vi "speedcontrol1old.vi"(11 "queue in":refnum<queue>) -> ()   [LabVIEW 2014]
uses:
  controls/UI Data.ctl
  controls/EncoderController.ctl
  <vilib>/Platform/TimedLoop/XDataNode/timing_clust.ctl
  <vilib>/Platform/TimedLoop/XDataNode/nitl_modes.ctl
  <vilib>/Platform/TimedLoop/XDataNode/wakeup.ctl
  controls/Control StateSam.ctl
  controls/Control ConfigurationSam.ctl
  <vilib>/Platform/TimedLoop/XDataNode/loadnilvce.vi
  <vilib>/addons/control/pid/pid.llb/PID (DBL Array).vi
  <vilib>/addons/control/pid/pid.llb/PID Percentage to EGU (DBL Array).vi
  <vilib>/platform/TimedLoop/XDataNode/XDataNode.xnode
  <vilib>/addons/control/pid/NI_PID_pid.lvlib
  <vilib>/Platform/TimedLoop/XDataNode/XDNodeRunTimeDep.lvlib
panel:
  out "Motor3Output":dbl
  out "Motor2Output":dbl
  out "Velocity3 RPM":dbl
  out "Velocity2 RPM":dbl
  out "Motor4Output":dbl
  out "Velocity4 RPM":dbl
  out "Motor1Output":dbl
  out "Velocity1 RPM":dbl
  # "0.8, 0. 0 is stable but theres a large offset\nsystem is slow to settle, increase Ti"
  # "Kp=2.04, Ti=0.15, Td=0.0375"
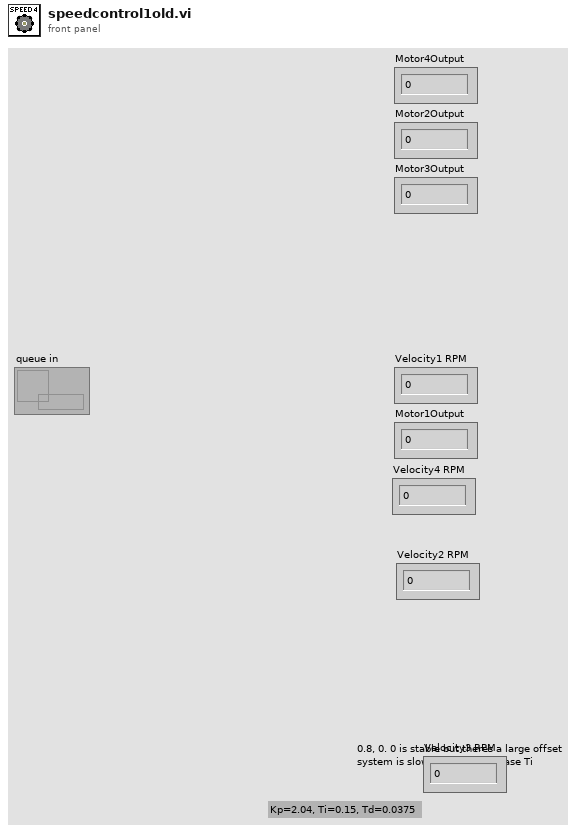
[diagram p1: front panel]
types:
  T1 = cluster{bool, "Tick Count(uSec)":u32, "Counter Value":i32, "x-y":i32}
  T2 = typedef "XDNodeRunTimeDep.lvlib/timing_clust.ctl" = cluster{"Expected End [f-1]":u64, "Actual End [f-1]":u64, "Finished Late? [f-1]":bool, "Expected End [i-1]":u64, "Actual End [i-1]":u64, "Finished Late? [i-1]":bool, "Expected Start [i]":u64, "Actual Start [i]":u64, "Expected Start [f]":u64, "Actual Start [f]":u64, "Source Name":string, "Structure Name":string, "Period":i64, "Deadline":i64, "Offset":i64, "Start":i64, "Priority":i32, "Timeout":i32, "Mode":T3, "Wakeup Reason":T4, "Error":errorcluster, "Source Type":string, "Secondary Source Type":string, "Global End Time":u64, "Global Start Time":u64, "Frame Duration":u64, "Iteration Duration":u64, "Assigned CPU":i32, "I/O Scan Engine Mode":u32}
  T3 = typedef "XDNodeRunTimeDep.lvlib/nitl_modes.ctl" = enum32{"No Change", "Process missed periods, maintain original phase", "Discard missed periods, maintain original phase", "Process missed periods, ignore original phase", "Discard missed periods, ignore original phase"}
  T4 = typedef "XDNodeRunTimeDep.lvlib/wakeup.ctl" = enum32{"Normal", "Aborted", "Asynchronous wakeup", "Timing source error", "Timed loop error", "Timeout"}
  T5 = typedef "EncoderController.ctl" = cluster{"Sample time (uS)":u32, "Reset":bool}
  T6 = typedef "EncoderIndicator.ctl" = cluster{"Position":dbl, "Velocity RPM":dbl, "Velocity RPS":dbl}
  T7 = typedef "Control StateSam.ctl" = enum16{"", "Control State (PID)", "Safe State"}
  T8 = typedef "Control ConfigurationSam.ctl" = cluster{"PID Gains":cluster{"proportional gain (Kc)":dbl, "integral gain (Kc*Ts/Ti)":dbl, "derivative gain (Kc*Td/Ts)":dbl}, "Output Range":cluster{"output high":dbl, "output low":dbl}}
  T9 = cluster{"proportional gain (Kc)":dbl, "integral gain (Kc*Ts/Ti)":dbl, "derivative gain (Kc*Td/Ts)":dbl}[]
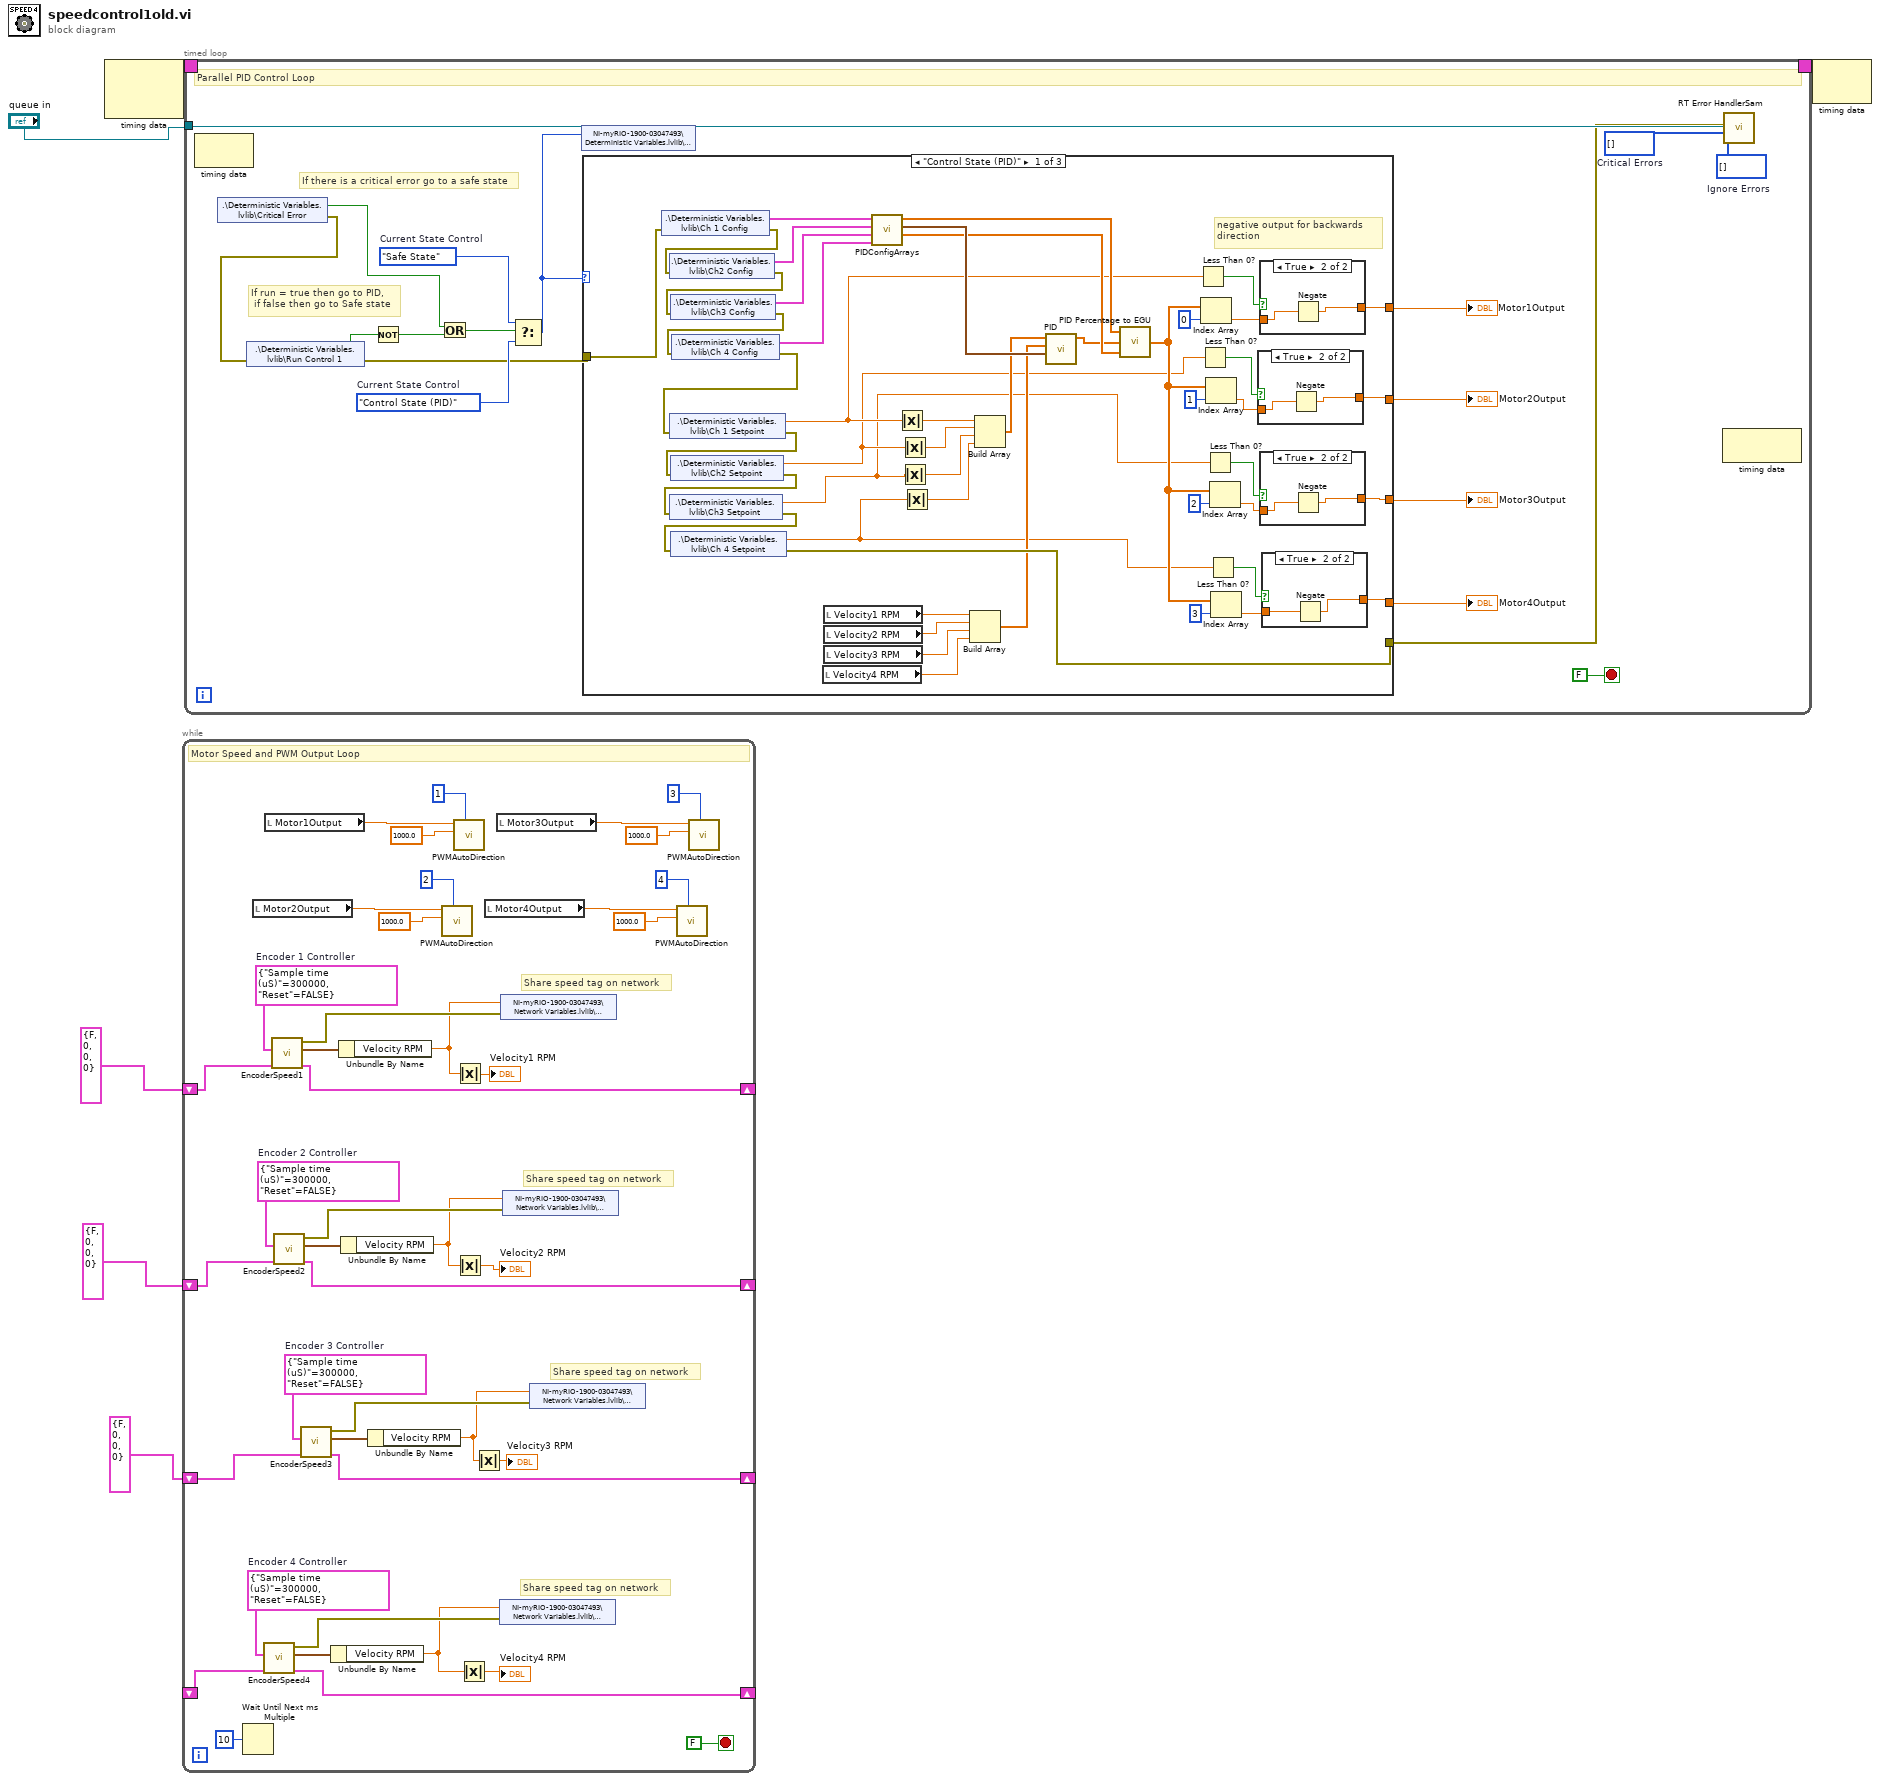
[diagram p0: block diagram]
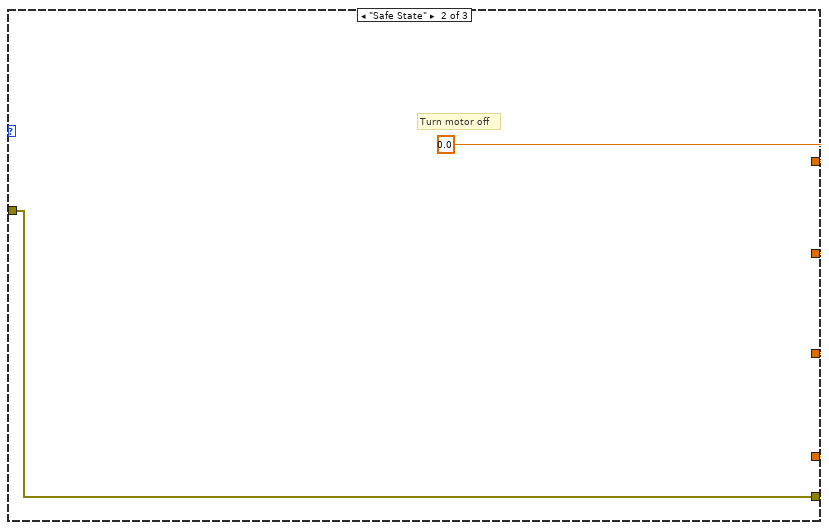
[diagram p6: hidden frame]
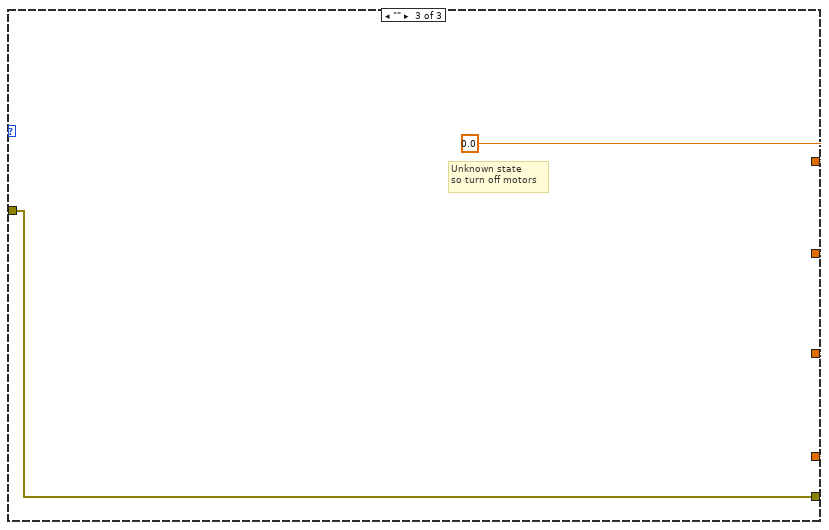
[diagram p7: hidden frame]
diagram:
  n1 = node-c288() -> (w6:T2)  [unwired: 2 in]
  n2 = while {
    shift-right: [w44] -> _
    shift-left: T1 {FALSE, "Tick Count(uSec)"=0, "Counter Value"=0, "x-y"=0} ("Cluster out") -> [w45]
    shift-right: [w34] -> _
    shift-left: _ -> [w35]
    shift-right: [w30] -> _
    shift-left: T1 {FALSE, "Tick Count(uSec)"=0, "Counter Value"=0, "x-y"=0} ("Cluster out") -> [w29]
    shift-right: [w21] -> _
    shift-left: T1 {FALSE, "Tick Count(uSec)"=0, "Counter Value"=0, "x-y"=0} ("Cluster out") -> [w22]
    stop <- FALSE stop-if-true
    w25 = T5 {"Sample time (uS)"=300000, "Reset"=FALSE}  # Encoder 3 Controller
    w26 = T5 {"Sample time (uS)"=300000, "Reset"=FALSE}  # Encoder 2 Controller
    w36 = T5 {"Sample time (uS)"=300000, "Reset"=FALSE}  # Encoder 4 Controller
    w48 = T5 {"Sample time (uS)"=300000, "Reset"=FALSE}  # Encoder 1 Controller
    # "Share speed tag on network"
    # "Share speed tag on network"
    # "Share speed tag on network"
    # "Share speed tag on network"
    # "Motor Speed and PWM Output Loop"
    n3 = Wait Until Next ms Multiple(millisecond multiple=u32 10) -> ()  [unwired: 1 out]
    n4 = local read "Motor2Output"() -> (w15:dbl)
    n5 = call "EncoderSpeed4.vi"("Cluster in"=w35, "Encoder 4 Controller"=w36) -> ("Cluster out"=w34:T1, "Encoder 4 Indicator"=w37:T6, "error out"=w38:errorcluster)  [unwired: 7 in]
    n6 = local read "Motor1Output"() -> (w41:dbl)
    n7 = call "EncoderSpeed1.vi"("Cluster in"=w45, "Encoder 1 Controller"=w48) -> ("Cluster out"=w44:T1, "Encoder 1 Indicator"=w47:T6, "error out"=w46:errorcluster)  [unwired: 7 in]
    n8 = call "EncoderSpeed2.vi"("Cluster in"=w29, "Encoder 2 Controller"=w26) -> ("Cluster out"=w30:T1, "Encoder 2 Indicator"=w27:T6, "error out"=w28:errorcluster)  [unwired: 7 in]
    n9 = call "EncoderSpeed3.vi"("Cluster in"=w22, "Encoder 3 Controller"=w25) -> ("Cluster out"=w21:T1, "Encoder 3 Indicator"=w24:T6, "error out"=w23:errorcluster)  [unwired: 7 in]
    n10 = Unbundle By Name(w37) -> ("Velocity RPM"=w7:dbl)
    n11 = Unbundle By Name(w47) -> ("Velocity RPM"=w13:dbl)
    n12 = Unbundle By Name(w27) -> ("Velocity RPM"=w12:dbl)
    n13 = Unbundle By Name(w24) -> ("Velocity RPM"=w10:dbl)
    n14 = call "PWMAutoDirection.vi"("Motor Select"=i8 2, "PWM Frequency"=1000.0, "DutyCycle"=w15) -> ()  [unwired: 8 in, 1 out]
    n15 = call "PWMAutoDirection.vi"("Motor Select"=i8 1, "PWM Frequency"=1000.0, "DutyCycle"=w41) -> ()  [unwired: 8 in, 1 out]
    n16 = Absolute Value(x=w13) -> (abs(x)=→"Velocity1 RPM":dbl)
    n17 = Absolute Value(x=w12) -> (abs(x)=→"Velocity2 RPM":dbl)
    n18 = Absolute Value(x=w7) -> (abs(x)=→"Velocity4 RPM":dbl)
    n19 = Absolute Value(x=w10) -> (abs(x)=→"Velocity3 RPM":dbl)
    n20 = local read "Motor4Output"() -> (w20:dbl)
    n21 = local read "Motor3Output"() -> (w31:dbl)
    n22 = shared-variable "NI-myRIO-1900-03047493\\Network Variables.lvlib\\SpeedMotor4"(w7, error in=w38) -> ()  [unwired: 1 out]
    n23 = shared-variable "NI-myRIO-1900-03047493\\Network Variables.lvlib\\SpeedMotor1"(w13, error in=w46) -> ()  [unwired: 1 out]
    n24 = shared-variable "NI-myRIO-1900-03047493\\Network Variables.lvlib\\SpeedMotor2"(w12, error in=w28) -> ()  [unwired: 1 out]
    n25 = shared-variable "NI-myRIO-1900-03047493\\Network Variables.lvlib\\SpeedMotor3"(w10, error in=w23) -> ()  [unwired: 1 out]
    n26 = call "PWMAutoDirection.vi"("Motor Select"=i8 4, "PWM Frequency"=1000.0, "DutyCycle"=w20) -> ()  [unwired: 8 in, 1 out]
    n27 = call "PWMAutoDirection.vi"("Motor Select"=i8 3, "PWM Frequency"=1000.0, "DutyCycle"=w31) -> ()  [unwired: 8 in, 1 out]
  }
  n28 = timed-loop {
    timing: w6 -> [_]
    timing-out: [_] -> w5
    tunnel: "queue in" -> [w54]
    stop <- FALSE stop-if-true
    w55 = i32[] []  # Critical Errors
    w56 = i32[] []  # Ignore Errors
    w63 = Control_StateSam."Control State (PID)"  # Current State Control
    w64 = Control_StateSam."Safe State"  # Current State Control
    # "If there is a critical error go to a safe state"
    # "If run = true then go to PID,\n if false then go to Safe state"
    # "Parallel PID Control Loop"
    n29 = node-c288() -> ()  [unwired: 1 in, 1 out]
    n30 = shared-variable ".\\Deterministic Variables.lvlib\\Critical Error"() -> (w60:bool, error out=w58:errorcluster)  [unwired: 1 in]
    n31 = shared-variable ".\\Deterministic Variables.lvlib\\Run Control 1"(error in=w58) -> (w65:bool, error out=w57:errorcluster)
    n32 = Not(x=w65) -> (.not. x?=w61:bool)
    n33 = Or(x=w60, y=w61) -> (x .or. y?=w59:bool)
    n34 = Select(t=w64, s=w59, f=w63) -> (s? t:f=w62:T7)
    n35 = shared-variable "NI-myRIO-1900-03047493\\Deterministic Variables.lvlib\\Control State"(w62) -> ()  [unwired: 1 in, 1 out]
    n36 = case shown="\"Control State (PID)\"" w62 {
      tunnel: [w86 w127 w129] -> w53
      tunnel: w57 -> [w97 w128 w130]
      tunnel: [w114 w128 w130] -> w52
      tunnel: [w80 w127 w129] -> w51
      tunnel: [w81 w127 w129] -> w50
      tunnel: [w82 w127 w129] -> w49
      frame "Control State (PID)" {
        # "negative output for backwards \ndirection"
        n37 = shared-variable ".\\Deterministic Variables.lvlib\\Ch 1 Config"(error in=w97) -> (w113:T8, error out=w96:errorcluster)
        n38 = shared-variable ".\\Deterministic Variables.lvlib\\Ch2 Config"(error in=w96) -> (w112:T8, error out=w95:errorcluster)
        n39 = shared-variable ".\\Deterministic Variables.lvlib\\Ch3 Config"(error in=w95) -> (w93:T8, error out=w94:errorcluster)
        n40 = shared-variable ".\\Deterministic Variables.lvlib\\Ch 4 Config"(error in=w94) -> (w92:T8, error out=w89:errorcluster)
        n41 = shared-variable ".\\Deterministic Variables.lvlib\\Ch 1 Setpoint"(error in=w89) -> (w74:dbl, error out=w100:errorcluster)
        n42 = shared-variable ".\\Deterministic Variables.lvlib\\Ch2 Setpoint"(error in=w100) -> (w72:dbl, error out=w99:errorcluster)
        n43 = shared-variable ".\\Deterministic Variables.lvlib\\Ch3 Setpoint"(error in=w99) -> (w68:dbl, error out=w98:errorcluster)
        n44 = shared-variable ".\\Deterministic Variables.lvlib\\Ch 4 Setpoint"(error in=w98) -> (w71:dbl, error out=w114:errorcluster)
        n45 = local read "Velocity4 RPM"() -> (w101:dbl)
        n46 = local read "Velocity1 RPM"() -> (w105:dbl)
        n47 = local read "Velocity2 RPM"() -> (w104:dbl)
        n48 = local read "Velocity3 RPM"() -> (w102:dbl)
        n49 = call "PIDConfigArrays.vi"("CH4"=w92, "CH3"=w93, "CH2"=w112, "CH1"=w113) -> ("OR Low array"=w109:dbl[], "OR High array"=w110:dbl[], "PID Gains array"=w111:T9)  [unwired: 5 in]
        n50 = Absolute Value(x=w74) -> (abs(x)=w73:dbl)
        n51 = Absolute Value(x=w72) -> (abs(x)=w69:dbl)
        n52 = Absolute Value(x=w68) -> (abs(x)=w67:dbl)
        n53 = Absolute Value(x=w71) -> (abs(x)=w70:dbl)
        n54 = Build Array(w105, w104, w102, w101) -> (w103:dbl[])
        n55 = Build Array(w73, w69, w67, w70) -> (w106:dbl[])
        n56 = call-poly <vilib>:"PID.vi"("PID gains"=w111, "process variable"=w103, "setpoint"=w106) -> ("output"=w75:dbl[])  [unwired: 7 in, 1 out]
        n57 = call-poly <vilib>:"PID Percentage to EGU.vi"("minimum (EGU)"=w109, "% span"=w75, "maximum (EGU)"=w110) -> ("output (EGU)"=w90:dbl[])  [unwired: 1 in]
        n58 = Less Than 0?(x=w74) -> (x < 0?=w88:bool)
        n59 = Less Than 0?(x=w72) -> (x < 0?=w78:bool)
        n60 = Index Array(array=w90, index=0) -> (element=w87:dbl)
        n61 = Less Than 0?(x=w68) -> (x < 0?=w77:bool)
        n62 = Index Array(array=w90, index=1) -> (element=w85:dbl)
        n63 = Less Than 0?(x=w71) -> (x < 0?=w76:bool)
        n64 = Index Array(array=w90, index=2) -> (element=w84:dbl)
        n65 = Index Array(array=w90, index=3) -> (element=w83:dbl)
        n66 = case shown="True" w78 {
          tunnel: w85 -> [w121 w123]
          tunnel: [w121 w122] -> w80
          frame False {
          }
          frame True {
            n67 = Negate(x=w123) -> (-x=w122:dbl)
          }
        }
        n68 = case shown="True" w88 {
          tunnel: w87 -> [w124 w126]
          tunnel: [w124 w125] -> w86
          frame False {
          }
          frame True {
            n69 = Negate(x=w126) -> (-x=w125:dbl)
          }
        }
        n70 = case shown="True" w77 {
          tunnel: w84 -> [w118 w120]
          tunnel: [w118 w119] -> w81
          frame False {
          }
          frame True {
            n71 = Negate(x=w120) -> (-x=w119:dbl)
          }
        }
        n72 = case shown="True" w76 {
          tunnel: w83 -> [w115 w117]
          tunnel: [w115 w116] -> w82
          frame False {
          }
          frame True {
            n73 = Negate(x=w117) -> (-x=w116:dbl)
          }
        }
      }
      frame "Safe State" {
        w127 = 0.0 ("output (EGU)")
        # "Turn motor off"
      }
      frame "" {
        w129 = 0.0 ("output (EGU)")
        # "Unknown state\nso turn off motors"
      }
    }
    "Motor1Output" <- w53
    "Motor4Output" <- w49
    "Motor2Output" <- w51
    "Motor3Output" <- w50
    n74 = node-c288() -> ()  [unwired: 1 in, 1 out]
    n75 = call "RT Error HandlerSam.vi"("Ignore Errors"=w56, "Critical Errors"=w55, "error to process"=w52, "queue in"=w54) -> ()  [unwired: 7 in, 1 out]
  }
  n76 = node-c288(w5) -> ()  [unwired: 1 out]
